vi "Configure Measurement Characteristics (Phase Noise).vi"(0 "VISA resource name":refnum<visa-resource-name>, 1 "Measurement Quality (1: Normal)":u16(ring)=1 items=["Fast", "Normal"], 5 "Frequency Band (3: Band 4)":u16(ring)=3 items=["Band 1 (10E6 to 41E6 Hz)", "Band 2 (39E6 to 101E6 Hz)", "Band 3 (99E6 to 1.5E9 Hz)", "Band 4 (250E6 to 7E9 Hz)", "Band 5 (3E9 to 10E9 Hz)", "Band 6 (9E9 to 26.5E9 Hz)"], 7 "Enable Carrier Search (Disable)":bool, 9 "Manual Nominal Frequency (3E9 Hz)":dbl=3000000000.0 format="%^#_9g", 11 "error in (no error)":errorcluster, 12 "Capture Range (0: Normal)":u16(ring) items=["Normal", "Wide"]) -> (4 "VISA resource name out":refnum<visa-resource-name>, 15 "error out":errorcluster)   [LabVIEW 2011, in "Agilent E5052X.lvlib"]
doc: "Configures initial settings for Phase Noise measurement. \n\n<b>Note: </b>\n\nThis VI must be called first before calling \"Configure Measurement(Phase Noise)\" VI."
uses:
  Agilent E5052X.lvlib
panel:
  # "Input Frequency Setting"
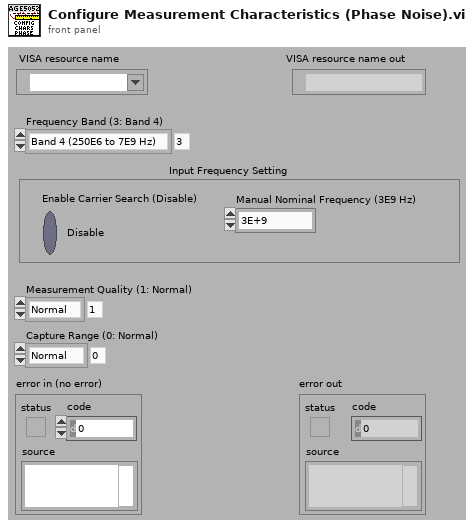
[diagram p1: front panel]
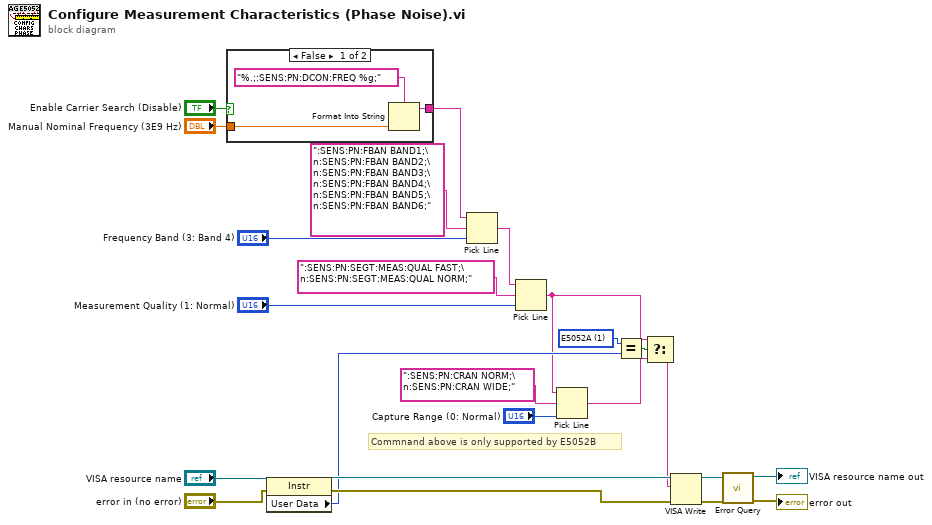
[diagram p0: block diagram]
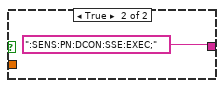
[diagram p2: hidden frame]
diagram:
  w4 = u16 1 items=["E5052B", "E5052A"] ("Ring")
  # "Commnand above is only supported by E5052B"
  n1 = case shown="False" "Enable Carrier Search (Disable)" {
    tunnel: "Manual Nominal Frequency (3E9 Hz)" -> [w27 _]
    tunnel: [w25 ":SENS:PN:DCON:SSE:EXEC;" ("write buffer")] -> w12
    frame False {
      n2 = Format Into String(format string="%.;:SENS:PN:DCON:FREQ %g;", w27) -> (resulting string=w25:string)  [unwired: 2 in, 1 out]
    }
    frame True {
    }
  }
  n3 = property class="Instr"(reference="VISA resource name", error in="error in (no error)") -> (reference out=w7:refnum<visa-resource-name>, error out=w6:errorcluster, "User Data"=w5:u32)
  n4 = Pick Line(string ("")=w12, multi-line string=":SENS:PN:FBAN BAND1;\n:SENS:PN:FBAN BAND2;\n:SENS:PN:FBAN BAND3;\n:SENS:PN:FBAN BAND4;\n:SENS:PN:FBAN BAND5;\n:SENS:PN:FBAN BAND6;", line index="Frequency Band (3: Band 4)") -> (output string=w11:string)
  n5 = Pick Line(string ("")=w11, multi-line string=":SENS:PN:SEGT:MEAS:QUAL FAST;\n:SENS:PN:SEGT:MEAS:QUAL NORM;", line index="Measurement Quality (1: Normal)") -> (output string=w3:string)
  n6 = Pick Line(string ("")=w3, multi-line string=":SENS:PN:CRAN NORM;\n:SENS:PN:CRAN WIDE;", line index="Capture Range (0: Normal)") -> (output string=w2:string)
  n7 = Equal?(x=w4, y=w5) -> (x = y?=w10:bool)
  n8 = Select(t=w3, s=w10, f=w2) -> (s? t:f=w1:string)
  n9 = VISA Write(VISA resource name=w7, write buffer=w1, error in (no error)=w6) -> (VISA resource name out=w22:refnum<visa-resource-name>, error out=w21:errorcluster)  [unwired: 1 out]
  n10 = call "Error Query.vi"("error in (no error)"=w21, "VISA resource name"=w22) -> ("error out"=→"error out":errorcluster, "VISA resource name out"=→"VISA resource name out":refnum<visa-resource-name>)  [unwired: 6 in, 2 out]
